vi "9604 String to Integer Overflow--error.vi"(7 "Type":T1(ring), 8 "error in":errorcluster, 11 "Integer String":string) -> (0 "error out":errorcluster)   [LabVIEW 2019, in "Electronic Datasheet.lvlib"]
uses:
  Electronic Datasheet.lvlib
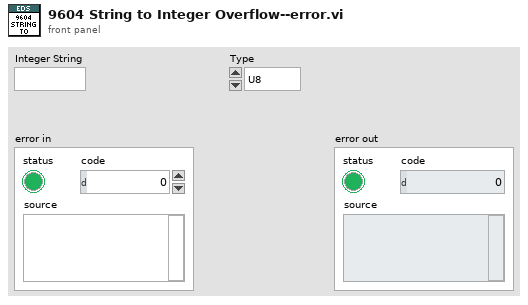
[diagram p1: front panel]
types:
  T1 = enum16{"U8", "U16", "U32", "I8", "I16", "I32", "I64", "U64"}
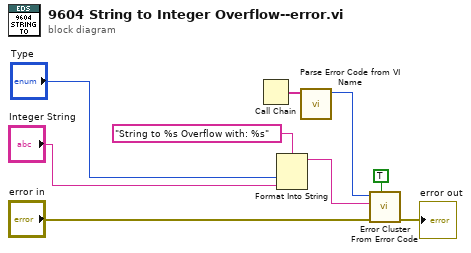
[diagram p0: block diagram]
diagram:
  n1 = Call Chain() -> (call chain=w2:string[])
  n2 = Format Into String(format string="String to %s Overflow with: %s" ("error message (\"\")"), "Type", "Integer String") -> (resulting string=w6:string)  [unwired: 2 in, 1 out]
  n3 = call "Parse Error Code from VI Name.vi"("Call Chain"=w2) -> ("Error Code"=w1:i32)  [unwired: 10 in]
  n4 = call <vilib>:"Error Cluster From Error Code.vi"("show call chain? (False)"=TRUE, "error in (no error)"="error in", "error message (\"\")"=w6, "error code (0)"=w1) -> ("error out"=→"error out":errorcluster)  [unwired: 5 in]
